vi "Recieve Idot Result utility.vi"(6 "Shots file":path=path "Z:/ShotHistory2014.txt", 7 "Log file folder":path=path "C:/Data/Shot Log.txt", 8 "error in (no error)":errorcluster, 10 "file path":path, 11 "Root Data Folder":path=path "C:/Data") -> (0 "error out":errorcluster, 3 "File Path output":path)   [LabVIEW 2015]
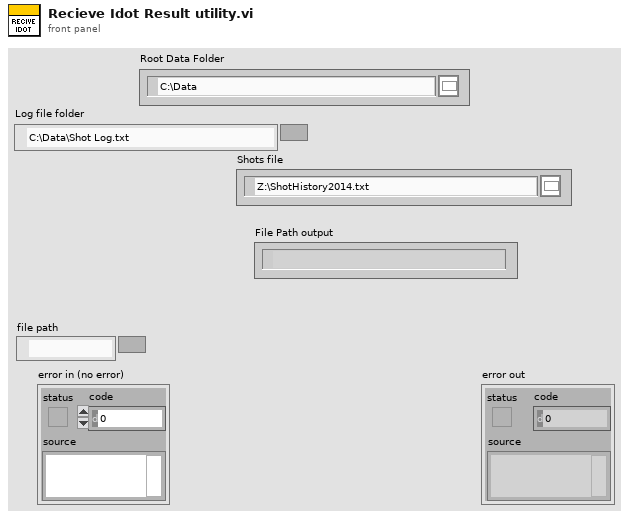
[diagram p1: front panel]
types:
  T1 = cluster{"file path":path, "Current time":timestamp, i32, dbl}
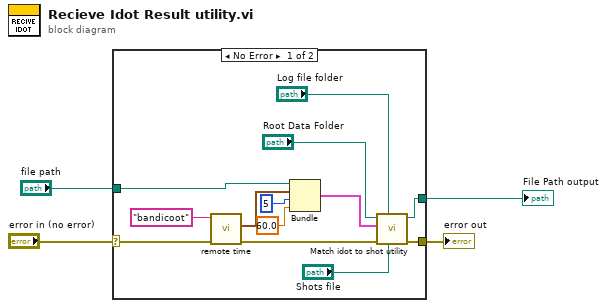
[diagram p0: block diagram]
diagram:
  n1 = case shown="No Error" "error in (no error)" {
    selector: "error in (no error)" -> [w17 w19]
    tunnel: [w8 w19] -> w3
    tunnel: [w6 w18] -> w2
    tunnel: "file path" -> [w5 w18]
    frame No Error {
      n2 = call "remote time.vi"("Error In"=w17, "server"="bandicoot" ("command line")) -> ("Error Out"=w7:errorcluster, "Current time"=w13:timestamp)  [unwired: 6 in, 2 out]
      n3 = Bundle("file path"=w5, "Current time"=w13, 5, 60.0) -> (w12:T1)  [unwired: 1 in]
      n4 = call "Match idot to shot utility.vi"("Shots file"="Shots file", "Log file folder"="Log file folder", "error in (no error)"=w7, "Idot match record"=w12, "Root Data Folder"="Root Data Folder") -> ("error out"=w8:errorcluster, "File output"=w6:path)  [unwired: 5 in]
    }
    frame Error {
    }
  }
  "error out" <- w3
  "File Path output" <- w2
